vi "Theta 1.vi"(5 "XYZ_60":dbl[](array[numeric])=[0.0, 0.0, 0.0], 7 "XYZ_0":dbl[](array[numeric])=[0.0, 0.0, 0.0], 9 "theta 2":dbl, 10 "theta 0":dbl, 11 "6R Type 1 Serial Arm Class in":refnum<class "NI_Robotics_6R Type 1 Serial Arm Class.lvclass">) -> (1 "Valid":bool, 2 "theta 1":dbl, 3 "6R Type 1 Serial Arm Class out":refnum<class "NI_Robotics_6R Type 1 Serial Arm Class.lvclass">)   [LabVIEW 2017, in "NI_Robotics_6R Type 1 Serial Arm Class.lvclass"]
uses:
  <vilib>/robotics/Kinematics/Analytical/6R/Type 1/NI_Robotics_6R Type 1 Serial Arm Class.lvclass
  c:/Program Files (x86)/National Instruments/LabVIEW 2017/vi.lib/robotics/Kinematics/Analytical/Generic/NI_Robotics_Analytical Serial Arm Class.lvclass
  <vilib>/Analysis/7linalg.llb/Solve Linear Equations (single right hand).vi
  <vilib>/Analysis/baseanly.llb/Solve Linear Equations By Cholesky.vi
  <vilib>/Analysis/baseanly.llb/Real Matrix to Compact Array.vi
  <vilib>/Analysis/baseanly.llb/Real Compact Tri-Matrix Linear Eqs.vi
  <vilib>/Analysis/7linalg.llb/Solve Linear Eqs (General).vi
  <vilib>/Analysis/7linalg.llb/Solve Linear Eqs (Gen, single right hand).vi
  <vilib>/Analysis/NI_AALPro.lvlib
  <vilib>/robotics/Kinematics/Analytical/Generic/NI_Robotics_Analytical Serial Arm Class.lvclass
panel:
  out "output array":dbl[][](array[numeric])
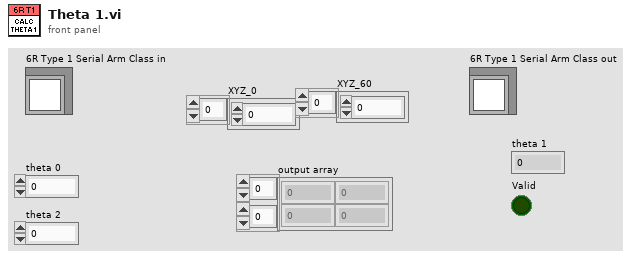
[diagram p1: front panel]
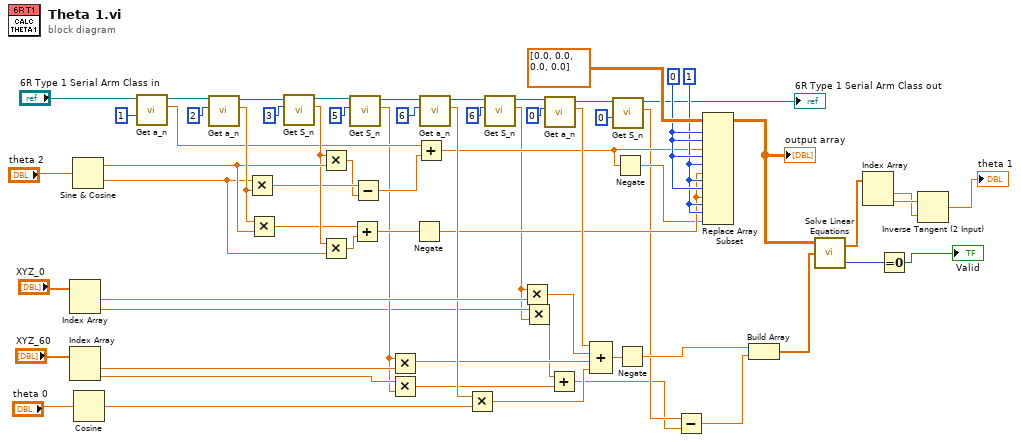
[diagram p0: block diagram]
diagram:
  w25 = 1 ("disabled index (col)")
  w26 = 0 ("index (row)")
  n1 = Index Array(array="XYZ_0") -> (element #1=w41:dbl, element #2=w15:dbl)  [unwired: 2 in]
  n2 = Index Array(array="XYZ_60") -> (element #1=w44:dbl, element #2=w17:dbl)  [unwired: 2 in]
  n3 = Sine & Cosine(0:"theta 2") -> (1:w52:dbl, 2:w50:dbl)
  n4 = Cosine(x="theta 0") -> (cos(x)=w39:dbl)
  n5 = call <vilib>:"Get a_n.vi"("n"=1, "Analytical Serial Arm Class in"="6R Type 1 Serial Arm Class in") -> ("a_n"=w28:dbl, "Analytical Serial Arm Class out"=w59:refnum<class "NI_Robotics_6R Type 1 Serial Arm Class.lvclass">)  [unwired: 8 in]
  n6 = call <vilib>:"Get a_n.vi"("n"=2, "Analytical Serial Arm Class in"=w59) -> ("a_n"=w53:dbl, "Analytical Serial Arm Class out"=w58:refnum<class "NI_Robotics_6R Type 1 Serial Arm Class.lvclass">)  [unwired: 8 in]
  n7 = Multiply(x=w50, y=w53) -> (x*y=w30:dbl)
  n8 = Multiply(x=w53, y=w52) -> (x*y=w48:dbl)
  n9 = call <vilib>:"Get S_n.vi"("n"=3, "Analytical Serial Arm Class in"=w58) -> ("S_n"=w51:dbl, "Analytical Serial Arm Class out"=w57:refnum<class "NI_Robotics_6R Type 1 Serial Arm Class.lvclass">)  [unwired: 8 in]
  n10 = Multiply(x=w51, y=w52) -> (x*y=w29:dbl)
  n11 = Multiply(x=w51, y=w50) -> (x*y=w49:dbl)
  n12 = call <vilib>:"Get S_n.vi"("n"=5, "Analytical Serial Arm Class in"=w57) -> ("S_n"=w16:dbl, "Analytical Serial Arm Class out"=w56:refnum<class "NI_Robotics_6R Type 1 Serial Arm Class.lvclass">)  [unwired: 8 in]
  n13 = Add(x=w48, y=w49) -> (x+y=w47:dbl)
  n14 = Subtract(x=w30, y=w29) -> (x-y=w31:dbl)
  n15 = Multiply(x=w16, y=w44) -> (x*y=w37:dbl)
  n16 = Multiply(x=w17, y=w16) -> (x*y=w13:dbl)
  n17 = Negate(x=w47) -> (-x=w23:dbl)
  n18 = Add(x=w28, y=w31) -> (x+y=w24:dbl)
  n19 = call <vilib>:"Get a_n.vi"("n"=6, "Analytical Serial Arm Class in"=w56) -> ("a_n"=w40:dbl, "Analytical Serial Arm Class out"=w43:refnum<class "NI_Robotics_6R Type 1 Serial Arm Class.lvclass">)  [unwired: 8 in]
  n20 = Multiply(x=w40, y=w39) -> (x*y=w36:dbl)
  n21 = call <vilib>:"Get S_n.vi"("n"=6, "Analytical Serial Arm Class in"=w43) -> ("S_n"=w14:dbl, "Analytical Serial Arm Class out"=w34:refnum<class "NI_Robotics_6R Type 1 Serial Arm Class.lvclass">)  [unwired: 8 in]
  n22 = Multiply(x=w14, y=w41) -> (x*y=w38:dbl)
  n23 = Multiply(x=w15, y=w14) -> (x*y=w12:dbl)
  n24 = call <vilib>:"Get a_n.vi"("n"=0, "Analytical Serial Arm Class in"=w34) -> ("a_n"=w32:dbl, "Analytical Serial Arm Class out"=w20:refnum<class "NI_Robotics_6R Type 1 Serial Arm Class.lvclass">)  [unwired: 8 in]
  n25 = Add(x=w12, y=w13) -> (x+y=w11:dbl)
  n26 = Compound Arithmetic op=ADD(w32, w38, w37, w36) -> (w35:dbl)
  n27 = call <vilib>:"Get S_n.vi"("n"=0, "Analytical Serial Arm Class in"=w20) -> ("S_n"=w18:dbl, "Analytical Serial Arm Class out"=→"6R Type 1 Serial Arm Class out":refnum<class "NI_Robotics_6R Type 1 Serial Arm Class.lvclass">)  [unwired: 8 in]
  n28 = Negate(x=w24) -> (-x=w22:dbl)
  n29 = Negate(x=w35) -> (-x=w21:dbl)
  n30 = Subtract(x=w18, y=w11) -> (x-y=w10:dbl)
  n31 = Replace Array Subset(array=dbl[][] [[0.0, 0.0], [0.0, 0.0]], new element #1=w24, index (row) #1=w26, index (col) #1=w26, new element #2=w23, index (row) #2=w26, index (col) #2=w25, new element #3=w23, index (row) #3=w25, index (col) #3=w26, new element #4=w22, index (row) #4=w25, index (col) #4=w25) -> (w9:dbl[][])
  "output array" <- w9
  n32 = Build Array(w21, w10) -> (w8:dbl[])
  n33 = call-poly <vilib>:"Solve Linear Equations.vi"("Known Vector"=w8, "Input Matrix"=w9) -> ("error"=w7:i32, "Solution Vector"=w4:dbl[])  [unwired: 1 in]
  n34 = Index Array(array=w4) -> (element #1=w2:dbl, element #2=w3:dbl)  [unwired: 2 in]
  n35 = Equal To 0?(x=w7) -> (x = 0?=→"Valid":bool)
  n36 = Inverse Tangent (2 Input)(1:w2, 2:w3) -> (0:→"theta 1":dbl)
